vi "HXG2_PIDs_Array.vi"(0 "Calculated Values":T3, 1 "PID Cluster":T7, 2 "Evap Target Delta (-°F) 2":cluster{"m":dbl, "b":dbl}={"m"=0.2667, "b"=7.333}, 3 "AIR-LIQ Cluster":T4 {"Liq Cluster"."Liq TEMP %" min=0.0 max=100.0 step=1.0 format="%#.1f"; "Liq Cluster"."Liq FLOW %" min=0.0 max=100.0 step=1.0 format="%#.1f"; "Liq Cluster"."TLiq °F" min=40.0 max=180.0 step=1.0 format="%#.1f"; "Liq Cluster"."Mdot lbm/hr" min=0.0 max=1000.0 step=1.0 format="%#.1f"; "Air Cluster"."Air TEMP %" min=0.0 max=100.0 step=1.0 format="%#.1f"; "Air Cluster"."Air FLOW %" min=0.0 max=100.0 step=1.0 format="%#.1f"; "Air Cluster"."Tair  °F" min=-5.0 max=100.0 step=1.0 format="%#.1f"; "Air Cluster"."CFMs" min=0.0 max=200.0 step=1.0 format="%#.1f"}, 4 "Tank Target Delta (+°F)":dbl, 5 "error in (no error)":errorcluster, 6 "Analog In":T2, 7 "PID Ctrls":T1) -> (14 "PID Ctrls Out":T1, 19 "error out":errorcluster)   [LabVIEW 2012]
uses:
  Controls/HXG2_PIDctrlsOUT.ctl
  Controls/HXG2_PIDCluster.ctl
  Controls/HXG2_PIDon-off.ctl
  PID/HXG2_Horizontal PID Control.ctl
  PID/HXG2_Horizontal Reset Control.ctl
  Controls/HXG2_AirGly-Cluster.ctl
  Controls/UI/HXG2_UI_ControlSetAir.ctl
  Controls/UI/HXG2_UI_ControlSetGly.ctl
  Controls/HXG2_Calculated.ctl
  Controls/HXG2_AnalogIn.ctl
  Modules/EnableAirGly/HXG2enable.ctl
  Controls/UI/HXG2_NumDisplayLarge.ctl
  <vilib>/addons/control/pid/pid.llb/PID Advanced (DBL Array).vi
  <vilib>/addons/control/pid/pid.llb/PID Derivative Action Buffered (DBL Array).vi
  <vilib>/addons/control/pid/pid.llb/PID Get Advanced Error (DBL Array).vi
  <vilib>/addons/control/pid/pid.llb/PID Integral Action Buffered (DBL Array).vi
  <vilib>/addons/control/pid/pid.llb/PID Resize 1D Array.vi
  <vilib>/addons/control/pid/pid.llb/PID Get Advanced Error (DBL).vi
  <vilib>/addons/control/pid/pid.llb/PID Control Input Filter (DBL).vi
  <vilib>/addons/control/pid/pid.llb/PID Gain Schedule (DBL).vi
  <vilib>/addons/control/pid/pid.llb/PID Structure Conversion (DBL).vi
  <vilib>/addons/control/pid/pid.llb/PID Parameter Manager (DBL Array).vi
  <vilib>/addons/control/pid/NI_PID_pid.lvlib
panel:
  out "index out 2":i32
  out "index out":i32
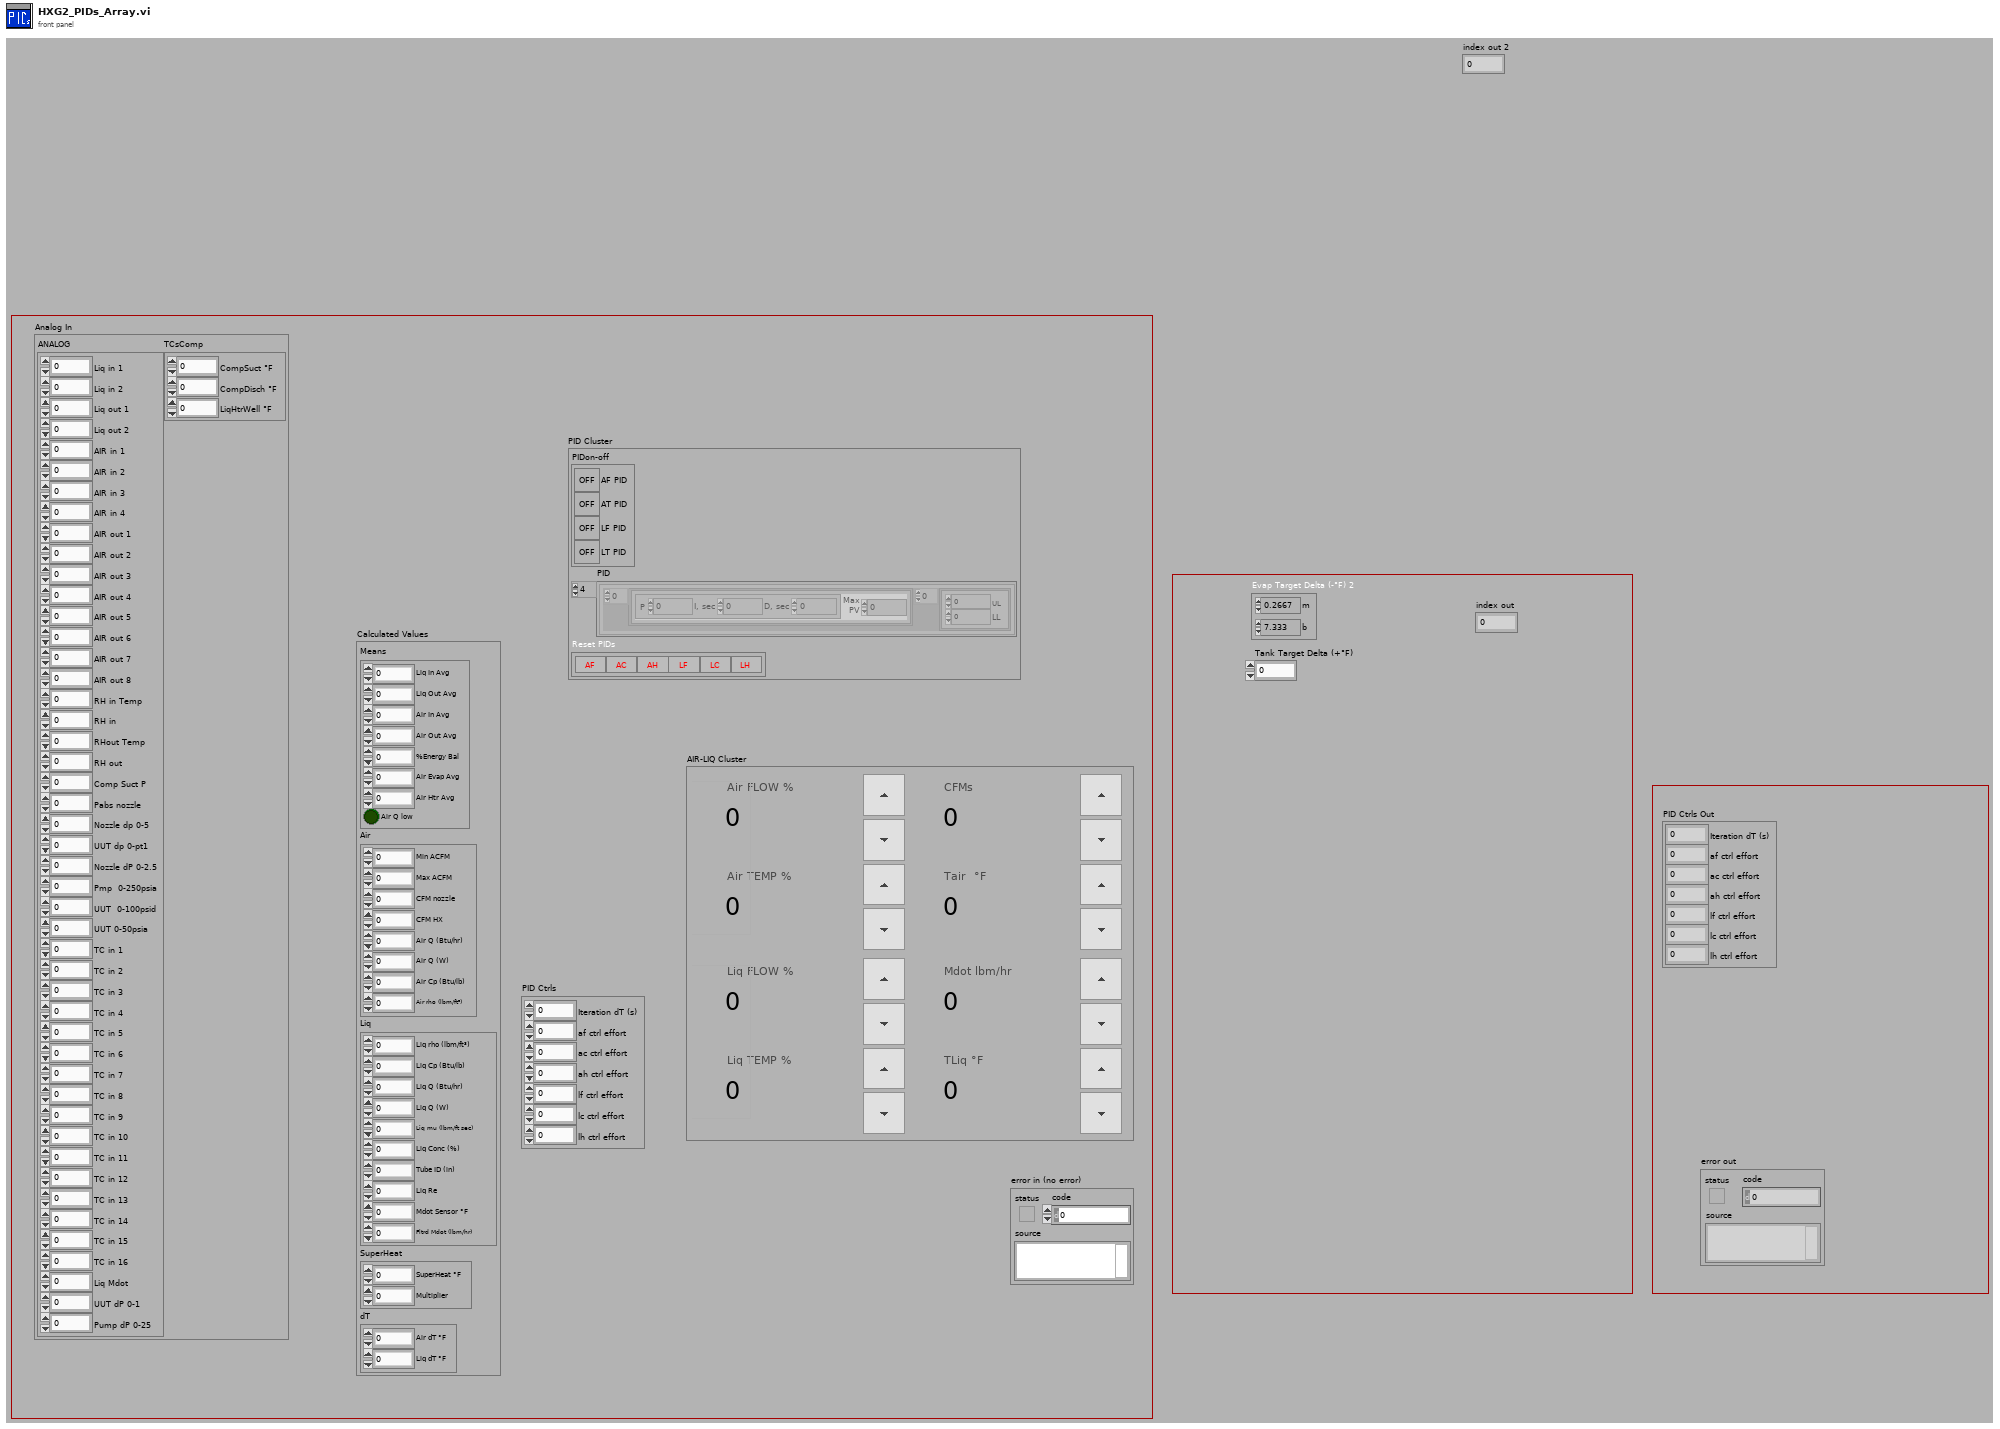
[diagram p1: front panel]
types:
  T1 = typedef "HXG2_PIDctrlsOUT.ctl" = cluster{"Iteration dT (s)":dbl, "af ctrl effort":dbl, "ac ctrl effort":dbl, "ah ctrl effort":dbl, "lf ctrl effort":dbl, "lc ctrl effort":dbl, "lh ctrl effort":dbl}
  T2 = typedef "HXG2_AnalogIn.ctl" = cluster{"ANALOG":cluster{"Liq in 1":dbl, "Liq in 2":dbl, "Liq out 1":dbl, "Liq out 2":dbl, "AIR in 1":dbl, "AIR in 2":dbl, "AIR in 3":dbl, "AIR in 4":dbl, "AIR out 1":dbl, "AIR out 2":dbl, "AIR out 3":dbl, "AIR out 4":dbl, "AIR out 5":dbl, "AIR out 6":dbl, "AIR out 7":dbl, "AIR out 8":dbl, "RH in Temp":dbl, "RH in":dbl, "RHout Temp":dbl, "RH out":dbl, "Comp Suct P":dbl, "Pabs nozzle":dbl, "Nozzle dp 0-5":dbl, "UUT dp 0-pt1":dbl, "Nozzle dP 0-2.5":dbl, "Pmp  0-250psia":dbl, "UUT  0-100psid":dbl, "UUT 0-50psia":dbl, "TC in 1":dbl, "TC in 2":dbl, "TC in 3":dbl, "TC in 4":dbl, "TC in 5":dbl, "TC in 6":dbl, "TC in 7":dbl, "TC in 8":dbl, "TC in 9":dbl, "TC in 10":dbl, "TC in 11":dbl, "TC in 12":dbl, "TC in 13":dbl, "TC in 14":dbl, "TC in 15":dbl, "TC in 16":dbl, "Liq Mdot":dbl, "UUT dP 0-1":dbl, "Pump dP 0-25":dbl}, "TCsComp":cluster{"CompSuct °F  ":dbl, "CompDisch °F":dbl, "LiqHtrWell °F":dbl}}
  T3 = typedef "HXG2_Calculated.ctl" = cluster{"Means":cluster{"Liq In Avg":dbl, "Liq Out Avg":dbl, "Air In Avg":dbl, "Air Out Avg":dbl, "%Energy Bal":dbl, "Air Evap Avg":dbl, "Air Htr Avg":dbl, "Air Q low":bool}, "Air":cluster{"Min ACFM":dbl, "Max ACFM":dbl, "CFM nozzle":dbl, "CFM HX":dbl, "Air Q (Btu/hr)":dbl, "Air Q (W)":dbl, "Air Cp (Btu/lb)":dbl, "Air rho (lbm/ft³)":dbl}, "Liq":cluster{"Liq rho (lbm/ft³)":dbl, "Liq Cp (Btu/lb)":dbl, "Liq Q (Btu/hr)":dbl, "Liq Q (W)":dbl, "Liq mu (lbm/ft sec)":dbl, "Liq Conc (%)":dbl, "Tube ID (in)":dbl, "Liq Re":dbl, "Mdot Sensor °F":dbl, "Fltrd Mdot (lbm/hr)":dbl}, "SuperHeat":cluster{"SuperHeat °F":dbl, "Multiplier":dbl}, "dT":cluster{"Air dT °F":dbl, "Liq dT °F":dbl}}
  T4 = typedef "HXG2_AirGly-Cluster.ctl" = cluster{"Air Cluster":T5, "Liq Cluster":T6}
  T5 = typedef "HXG2_UI_ControlSetAir.ctl" = cluster{"Air FLOW %":dbl, "Air TEMP % ":dbl, "CFMs":dbl, "Tair  °F":dbl}
  T6 = typedef "HXG2_UI_ControlSetGly.ctl" = cluster{"Liq FLOW %":dbl, "Liq TEMP % ":dbl, "Mdot lbm/hr":dbl, "TLiq °F":dbl}
  T7 = typedef "HXG2_PIDCluster.ctl" = cluster{"PIDon-off ":T8, "PID":T9, "Reset PIDs":T10}
  T8 = typedef "HXG2_PIDon-off.ctl" = cluster{"AF PID":bool, "AT PID":bool, "LF PID":bool, "LT PID":bool}
  T9 = typedef "HXG2_Horizontal PID Control.ctl" = cluster{"GainsArray":cluster{"Gains 2":cluster{"P":dbl, "I, sec":dbl, "D, sec":dbl}, "Max\nPV":dbl}[], "UL-LL Array":cluster{"UL":dbl, "LL  ":dbl}[]}[]
  T10 = typedef "HXG2_Horizontal Reset Control.ctl" = cluster{"AF":bool, "AC":bool, "AH":bool, "LF":bool, "LC":bool, "LH":bool}
  T11 = cluster{"setpoint high":dbl, "setpoint low":dbl}[]
  T12 = typedef "HXG2enable.ctl" = enum16{"Write Refs", "Write", "Pass"}
  T13 = enum16{"Academic (Standard)", "Parallel", "Series"}
  T14 = typedef "HXG2_NumDisplayLarge.ctl" = dbl
  T15 = cluster{"Gains 2":cluster{"P":dbl, "I, sec":dbl, "D, sec":dbl}, "Max\nPV":dbl}[]
  T16 = cluster{"proportional gain (Kc)":dbl, "integral time (Ti, min)":dbl, "derivative time (Td, min)":dbl}
  T17 = cluster{"output[0]":dbl, "output[1]":dbl, "output[2]":dbl}
  T18 = cluster{"[0]":dbl, "[1]":dbl, "[2]":dbl, "[3]":dbl}
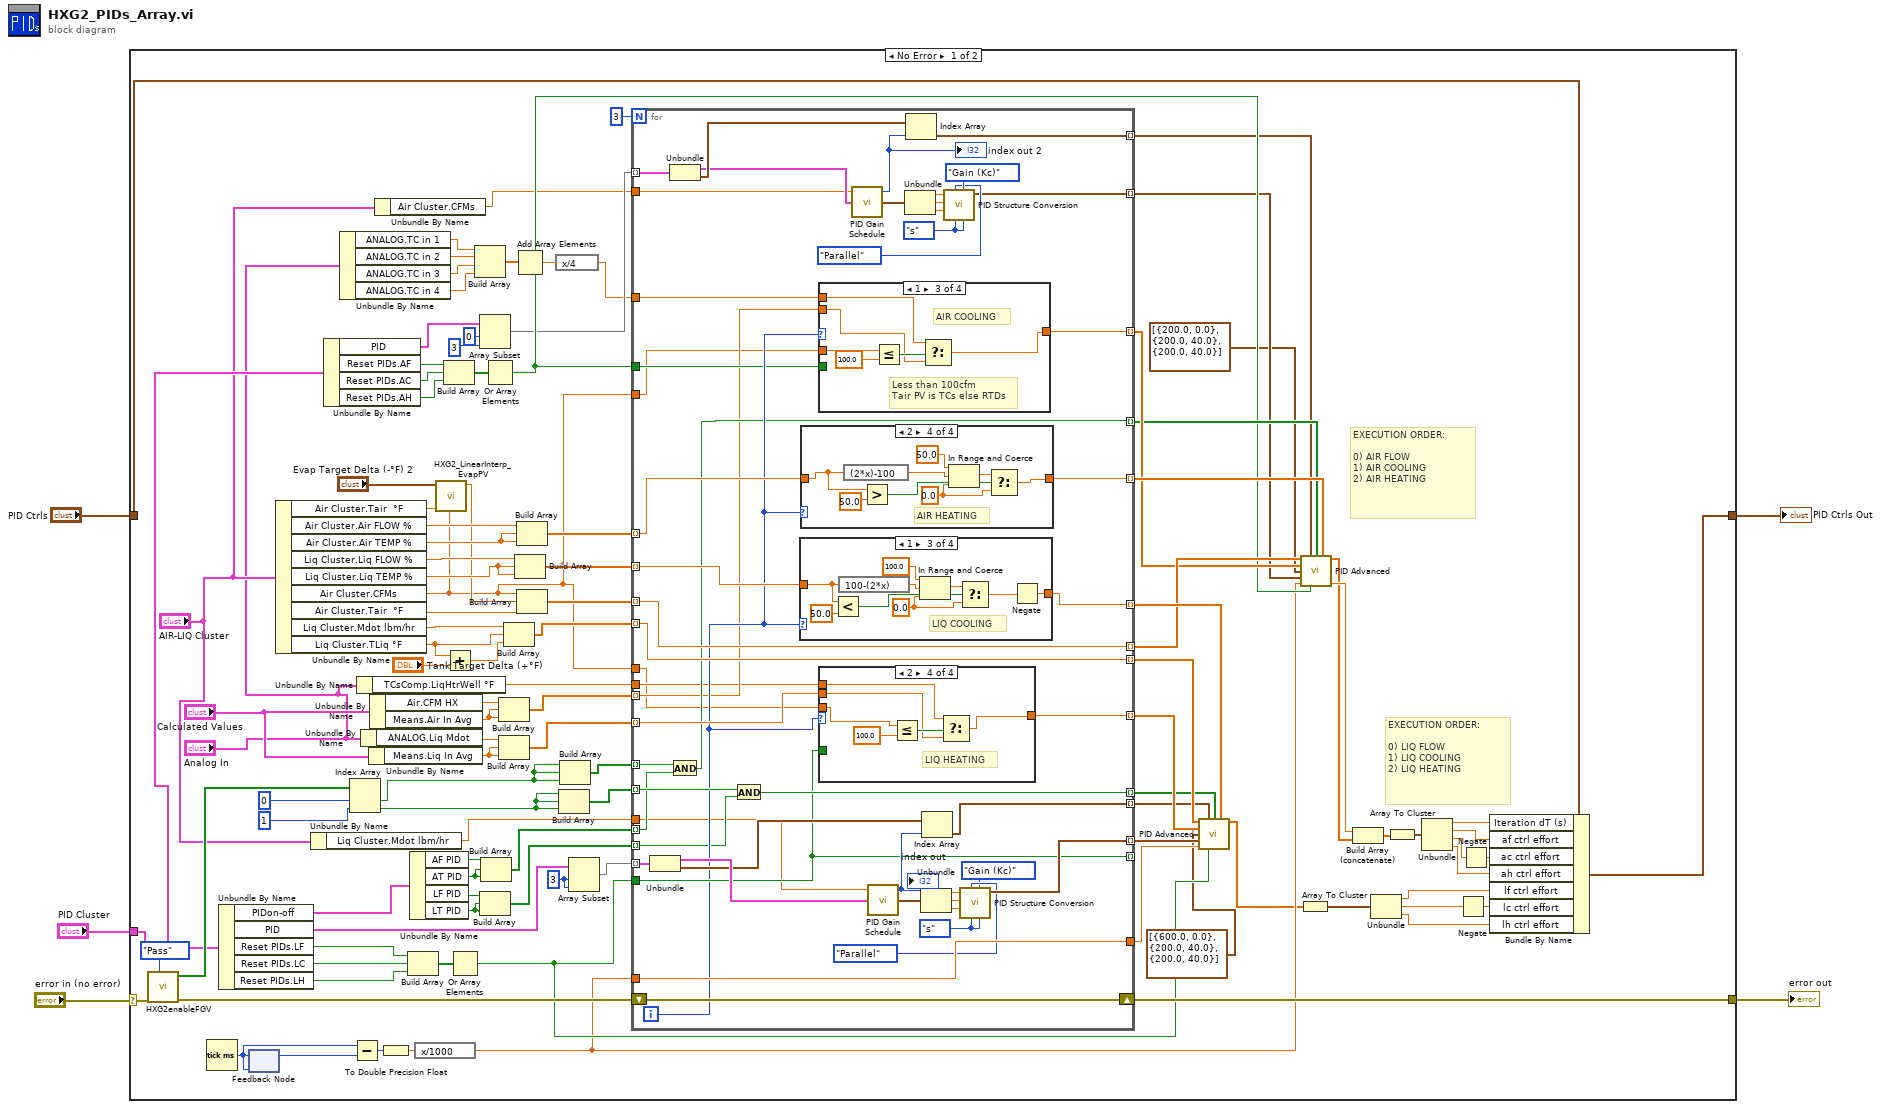
[diagram p0: block diagram]
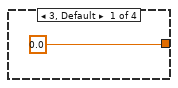
[diagram p2: hidden frame]
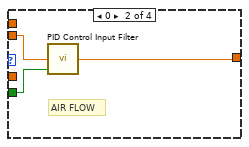
[diagram p3: hidden frame]
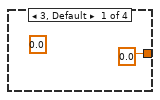
[diagram p5: hidden frame]
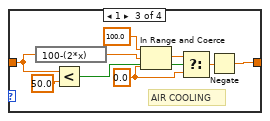
[diagram p7: hidden frame]
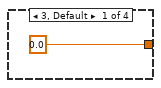
[diagram p8: hidden frame]
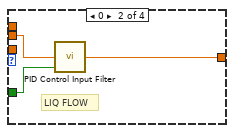
[diagram p9: hidden frame]
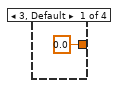
[diagram p11: hidden frame]
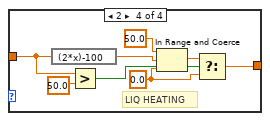
[diagram p13: hidden frame]
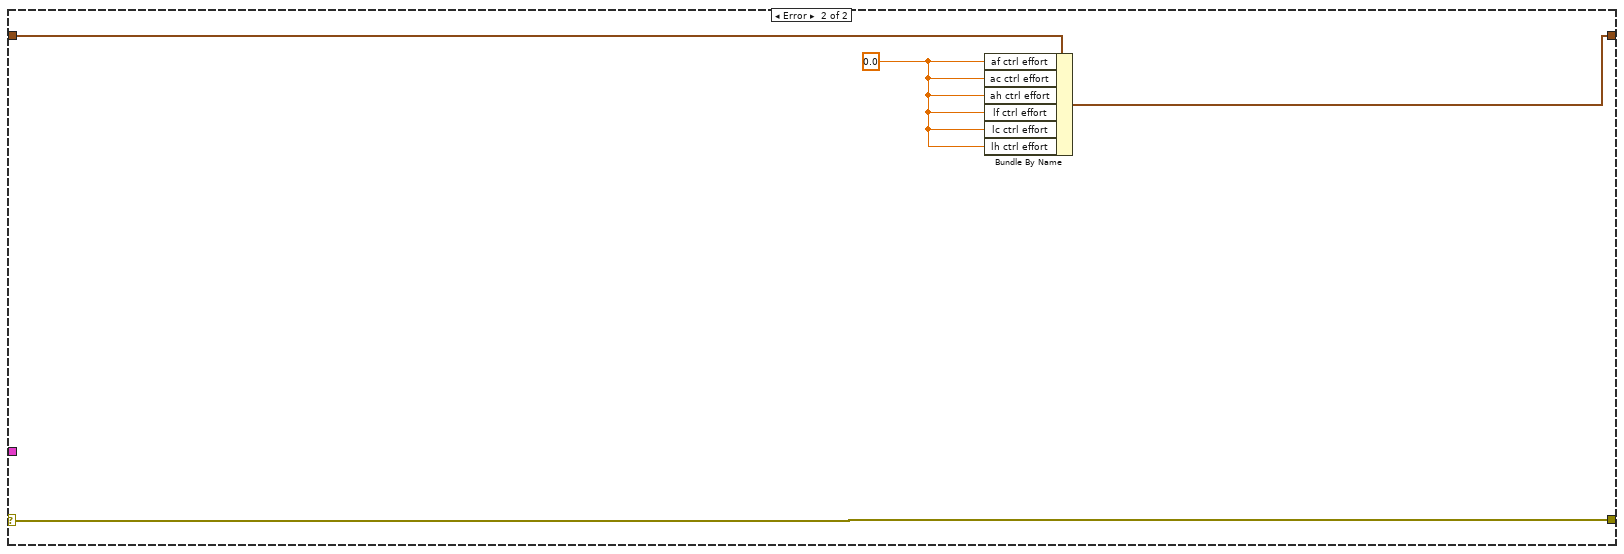
[diagram p14: hidden frame]
diagram:
  n1 = case shown="No Error" "error in (no error)" {
    selector: "error in (no error)" -> [w115 w232]
    tunnel: [w99 w232] -> w5
    tunnel: [w97 w230] -> w2
    tunnel: "PID Ctrls" -> [w98 w231]
    tunnel: "PID Cluster" -> [w61 _]
    frame No Error {
      w49 = 3 ("index")
      # "EXECUTION ORDER:\n\n0) AIR FLOW\n1) AIR COOLING\n2) AIR HEATING"
      # "EXECUTION ORDER:\n\n0) LIQ FLOW\n1) LIQ COOLING\n2) LIQ HEATING"
      n2 = call "HXG2enableFGV.vi"("ENABLE Ctrl"=HXG2enable."Pass", "error in (no error)"=w115) -> ("error out"=w100:errorcluster, "Air-Liq Out"=w102:bool[])  [unwired: 7 in, 1 out]
      n3 = Tick Count (ms)() -> (millisecond timer value=w108:u32)
      n4 = Unbundle By Name(w61) -> ("PIDon-off"=w94:T8, "PID"=w50:T9, "Reset PIDs.LF"=w56:bool, "Reset PIDs.LC"=w55:bool, "Reset PIDs.LH"=w54:bool)
      n5 = feedback #1(w108) -> (w106:u32)
      n6 = feedback-in #1(w108) -> ()
      n7 = Unbundle By Name("AIR-LIQ Cluster") -> ("Air Cluster.Tair  °F"=w8:dbl, "Air Cluster.Air FLOW %"=w84:dbl, "Air Cluster.Air TEMP %"=w83:dbl, "Liq Cluster.Liq FLOW %"=w112:dbl, "Liq Cluster.Liq TEMP %"=w111:dbl, "Air Cluster.CFMs"=w6:dbl, "Air Cluster.Tair  °F"=w15:dbl, "Liq Cluster.Mdot lbm/hr"=w26:dbl, "Liq Cluster.TLiq °F"=w13:dbl)
      n8 = Unbundle By Name("AIR-LIQ Cluster") -> ("Liq Cluster.Mdot lbm/hr"=w23:dbl)
      n9 = Unbundle By Name(w61) -> ("PID"=w46:T9, "Reset PIDs.AF"=w60:bool, "Reset PIDs.AC"=w59:bool, "Reset PIDs.AH"=w58:bool)
      n10 = Unbundle By Name("Analog In") -> ("ANALOG.TC in 1"=w22:dbl, "ANALOG.TC in 2"=w21:dbl, "ANALOG.TC in 3"=w20:dbl, "ANALOG.TC in 4"=w19:dbl)
      n11 = Index Array(array=w102, index #1=0 ("index"), index #2=1 ("index")) -> (element #1=w70:bool, element #2=w103:bool)
      n12 = Subtract(x=w108, y=w106) -> (x-y=w107:u32)
      n13 = Unbundle By Name("Analog In") -> ("TCsComp.LiqHtrWell °F"=w10:dbl)
      n14 = Unbundle By Name("Analog In") -> ("ANALOG.Liq Mdot"=w75:dbl)
      n15 = Unbundle By Name("Calculated Values") -> ("Means.Liq In Avg"=w74:dbl)
      n16 = Unbundle By Name("Calculated Values") -> ("Air.CFM HX"=w77:dbl, "Means.Air In Avg"=w76:dbl)
      n17 = Unbundle By Name("AIR-LIQ Cluster") -> ("Air Cluster.CFMs"=w25:dbl)
      n18 = To Double Precision Float(number=w107) -> (double precision float=w109:dbl)
      n19 = Build Array(w56, w55, w54) -> (w53:bool[])
      n20 = Unbundle By Name(w94) -> ("AF PID"=w66:bool, "AT PID"=w65:bool, "LF PID"=w67:bool, "LT PID"=w64:bool)
      n21 = expression code="x/1000"(w109) -> (w41:dbl)
      n22 = call "HXG2_LinearInterp_EvapPV.vi"("CFM"=w6, "Tair  °F"=w8, "Evap Target Delta (-°F) in"="Evap Target Delta (-°F) 2") -> ("Evap Target (F)"=w7:dbl)  [unwired: 8 in]
      n23 = Build Array(w60, w59, w58) -> (w57:bool[])
      n24 = Add(x=w13, y="Tank Target Delta (+°F)") -> (x+y=w12:dbl)
      n25 = Or Array Elements(Boolean array=w53) -> (logical OR=w52:bool)
      n26 = Build Array(w22, w21, w20, w19) -> (w18:dbl[])
      n27 = Array Subset(array=w46, index=0, length=3 ("index")) -> (w44:T9)
      n28 = Build Array(w67, w64, w64) -> (w63:bool[])
      n29 = Build Array(w66, w65, w65) -> (w62:bool[])
      n30 = Or Array Elements(Boolean array=w57) -> (logical OR=w51:bool)
      n31 = Build Array(w77, w76, w76) -> (w72:dbl[])
      n32 = Build Array(w75, w74, w74) -> (w73:dbl[])
      n33 = Build Array(w26, w13, w12) -> (w78:dbl[])
      n34 = Add Array Elements(numeric array=w18) -> (sum=w17:dbl)
      n35 = Build Array(w112, w111, w111) -> (w110:dbl[])
      n36 = Build Array(w84, w83, w83) -> (w82:dbl[])
      n37 = Build Array(w6, w7, w15) -> (w80:dbl[])
      n38 = expression code="x/4"(w17) -> (w16:dbl)
      n39 = Build Array(w103, w103, w103) -> (w101:bool[])
      n40 = Build Array(w70, w70, w70) -> (w69:bool[])
      n41 = Array Subset(array=w50, index=w49, length=w49) -> (w48:T9)
      n42 = for {
        N: 3 -> [_]
        tunnel: w63 -> [w140] mode=indexing
        tunnel: w73 -> [w159] mode=indexing
        tunnel: w78 -> [w155] mode=indexing
        tunnel: w110 -> [w165] mode=indexing
        tunnel: w41 -> [w150]
        tunnel: w101 -> [w168] mode=indexing
        tunnel: w48 -> [w167] mode=indexing
        shift-right: [w166] -> w99
        shift-left: w100 -> [w166]
        tunnel: w52 -> [w149]
        tunnel: [w155] -> w93 mode=indexing
        tunnel: [w154] -> w92 mode=indexing
        tunnel: [w153] -> w91 mode=indexing
        tunnel: [w152] -> w90 mode=indexing
        tunnel: [w146] -> w89 mode=indexing
        tunnel: [w151] -> w88 mode=indexing
        tunnel: [w150] -> w87
        tunnel: [w149] -> _ mode=indexing
        tunnel: w82 -> [w145] mode=indexing
        tunnel: [w144] -> w81 mode=indexing
        tunnel: w80 -> [w143] mode=indexing
        tunnel: [w143] -> w79 mode=indexing
        tunnel: w72 -> [w124] mode=indexing
        tunnel: [w142] -> w71 mode=indexing
        tunnel: w69 -> [w139] mode=indexing
        tunnel: [w138] -> w68 mode=indexing
        tunnel: w62 -> [w137] mode=indexing
        tunnel: w51 -> [w136]
        tunnel: w44 -> [w127] mode=indexing
        tunnel: [w123] -> w43 mode=indexing
        tunnel: [w122] -> w42 mode=indexing
        tunnel: w25 -> [w121]
        tunnel: w23 -> [w120]
        tunnel: w16 -> [w119]
        tunnel: w10 -> [w118]
        tunnel: w6 -> [w117]
        tunnel: w6 -> [w116]
        i -> [w141]
        w132 = enum16{"min", "s"}."s" ("integral unit")
        w160 = enum16{"min", "s"}."s" ("integral unit")
        n43 = Unbundle(w167) -> ("GainsArray"=w157:T15, "UL-LL Array"=w156:cluster{"UL":dbl, "LL  ":dbl}[])
        n44 = Unbundle(w127) -> ("GainsArray"=w125:T15, "UL-LL Array"=w126:cluster{"UL":dbl, "LL  ":dbl}[])
        n45 = And(x=w139, y=w137) -> (x .and. y?=w138:bool)
        n46 = And(x=w168, y=w140) -> (x .and. y?=w152:bool)
        n47 = case shown="1" w141 {
          tunnel: w165 -> [_ w211 w213 w223]
          tunnel: [0.0 ("Liq In Avg") w211 w212 w221] -> w153
          frame 3, Default {
          }
          frame 0 {
            # "LIQ FLOW"
          }
          frame 1 {
            w216 = T14 0.0 ("lower limit")
            # "LIQ COOLING"
            n48 = Less?(x=w213, y=T14 50.0) -> (x < y?=w215:bool)
            n49 = expression code="100-(2*x)"(w213) -> (w218:dbl)
            n50 = In Range and Coerce(upper limit=T14 100.0, x=w218, lower limit=w216) -> (coerced(x)=w219:T14)  [unwired: 1 out]
            n51 = Select(t=w219, s=w215, f=w216) -> (s? t:f=w220:T14)
            n52 = Negate(x=w220) -> (-x=w212:T14)
          }
          frame 2 {
            w228 = T14 0.0 ("lower limit")
            # "LIQ HEATING"
            n53 = expression code="(2*x)-100"(w223) -> (w226:dbl)
            n54 = Greater?(x=w223, y=T14 50.0) -> (0:w224:bool)
            n55 = In Range and Coerce(upper limit=T14 50.0, x=w226, lower limit=w228) -> (coerced(x)=w227:T14)  [unwired: 1 out]
            n56 = Select(t=w227, s=w224, f=w228) -> (s? t:f=w221:T14)
          }
        }
        n57 = case shown="2" w141 {
          tunnel: w145 -> [_ w181 w184 w193]
          tunnel: [0.0 ("Liq In Avg") w181 w182 w191] -> w144
          frame 3, Default {
            (unwired) 0.0 ("Liq In Avg")
          }
          frame 0 {
            # "AIR FLOW"
          }
          frame 1 {
            w186 = T14 0.0 ("lower limit")
            # "AIR COOLING"
            n58 = expression code="100-(2*x)"(w184) -> (w187:dbl)
            n59 = Less?(x=w184, y=T14 50.0) -> (x < y?=w185:bool)
            n60 = In Range and Coerce(upper limit=T14 100.0, x=w187, lower limit=w186) -> (coerced(x)=w188:T14)  [unwired: 1 out]
            n61 = Select(t=w188, s=w185, f=w186) -> (s? t:f=w190:T14)
            n62 = Negate(x=w190) -> (-x=w182:T14)
          }
          frame 2 {
            w198 = T14 0.0 ("lower limit")
            # "AIR HEATING"
            n63 = expression code="(2*x)-100"(w193) -> (w196:dbl)
            n64 = Greater?(x=w193, y=T14 50.0) -> (0:w194:bool)
            n65 = In Range and Coerce(upper limit=T14 50.0, x=w196, lower limit=w198) -> (coerced(x)=w197:T14)  [unwired: 1 out]
            n66 = Select(t=w197, s=w194, f=w198) -> (s? t:f=w191:T14)
          }
        }
        n67 = case shown="1" w141 {
          tunnel: w124 -> [_ w172 w175 w179]
          tunnel: [0.0 ("Liq In Avg") w171 w173 w179] -> w142
          tunnel: w136 -> [_ w170 _ _]
          tunnel: w119 -> [_ _ w174 _]
          tunnel: w117 -> [_ _ w178 _]
          frame 3, Default {
          }
          frame 0 {
            # "AIR FLOW"
            n68 = call-poly <vilib>:"PID Control Input Filter.vi"("reinitialize? (F)"=w170, "input"=w172) -> ("output"=w171:dbl)  [unwired: 3 in]
          }
          frame 1 {
            # "Less than 100cfm\nTair PV is TCs else RTDs"
            # "AIR COOLING"
            n69 = Less Or Equal?(x=w178, y=100.0) -> (x <= y?=w176:bool)
            n70 = Select(t=w174, s=w176, f=w175) -> (s? t:f=w173:dbl)
          }
          frame 2 {
            # "AIR HEATING"
          }
        }
        n71 = case shown="2" w141 {
          tunnel: w159 -> [_ w202 w203 w206]
          tunnel: [0.0 ("Liq In Avg") w200 w203 w204] -> w154
          tunnel: w149 -> [_ w201 _ _]
          tunnel: w118 -> [_ _ _ w205]
          tunnel: w116 -> [_ _ _ w207]
          frame 3, Default {
          }
          frame 0 {
            # "LIQ FLOW"
            n72 = call-poly <vilib>:"PID Control Input Filter.vi"("reinitialize? (F)"=w201, "input"=w202) -> ("output"=w200:dbl)  [unwired: 3 in]
          }
          frame 1 {
            # "LIQ COOLING"
          }
          frame 2 {
            # "LIQ HEATING"
            n73 = Less Or Equal?(x=w207, y=100.0) -> (x <= y?=w209:bool)
            n74 = Select(t=w205, s=w209, f=w206) -> (s? t:f=w204:dbl)
          }
        }
        n75 = call-poly <vilib>:"PID Gain Schedule.vi"("PID gain schedule"=w125, "gain scheduling value"=w121) -> ("PID gains out"=w128:T16, "index out"=w133:i32)  [unwired: 2 in]
        "index out 2" <- w133
        n76 = call-poly <vilib>:"PID Gain Schedule.vi"("PID gain schedule"=w157, "gain scheduling value"=w120) -> ("PID gains out"=w164:T16, "index out"=w158:i32)  [unwired: 2 in]
        "index out" <- w158
        n77 = Unbundle(w128) -> ("proportional gain (Kc)"=w129:dbl, "integral time (Ti, min)"=w130:dbl, "derivative time (Td, min)"=w131:dbl)
        n78 = Index Array(array=w126, index=w133) -> (element=w122:cluster{"UL":dbl, "LL  ":dbl})
        n79 = Unbundle(w164) -> ("proportional gain (Kc)"=w163:dbl, "integral time (Ti, min)"=w162:dbl, "derivative time (Td, min)"=w161:dbl)
        n80 = Index Array(array=w156, index=w158) -> (element=w146:cluster{"UL":dbl, "LL  ":dbl})
        n81 = call-poly <vilib>:"PID Structure Conversion.vi"("derivative unit"=w132, "proportional unit"=enum16{"Gain (Kc)", "Band (PB)"}."Gain (Kc)", "integral unit"=w132, "PID structure"=T13."Parallel", "derivative"=w131, "integral"=w130, "proportional"=w129) -> ("PID gains"=w123:T16)  [unwired: 4 in]
        n82 = call-poly <vilib>:"PID Structure Conversion.vi"("derivative unit"=w160, "proportional unit"=enum16{"Gain (Kc)", "Band (PB)"}."Gain (Kc)", "integral unit"=w160, "PID structure"=T13."Parallel", "derivative"=w161, "integral"=w162, "proportional"=w163) -> ("PID gains"=w151:T16)  [unwired: 4 in]
      }
      n83 = call-poly <vilib>:"PID Advanced.vi"("setpoint"=w93, "output range"=w89, "auto? (T)"=w90, "manual control"=w91, "process variable"=w92, "setpoint range"=T11 [{"setpoint high"=600.0, "setpoint low"=0.0}, {"setpoint high"=200.0, "setpoint low"=40.0}, {"setpoint high"=200.0, "setpoint low"=40.0}], "PID gains"=w88, "dt (s)"=w87, "reinitialize? (F)"=w52) -> ("output"=w40:dbl[])  [unwired: 5 in, 1 out]
      n84 = Array To Cluster(array=w40) -> (cluster=w96:T17)
      n85 = call-poly <vilib>:"PID Advanced.vi"("setpoint"=w79, "output range"=w42, "auto? (T)"=w68, "manual control"=w81, "process variable"=w71, "setpoint range"=T11 [{"setpoint high"=200.0, "setpoint low"=0.0}, {"setpoint high"=200.0, "setpoint low"=40.0}, {"setpoint high"=200.0, "setpoint low"=40.0}], "PID gains"=w43, "dt (s)"=w41, "reinitialize? (F)"=w51) -> ("output"=w35:dbl[], "dt out (s)"=w36:dbl)  [unwired: 5 in]
      n86 = Build Array (concatenate)(w36, w35) -> (w34:dbl[])
      n87 = Unbundle(w96) -> ("output[0]"=w39:dbl, "output[1]"=w38:dbl, "output[2]"=w37:dbl)
      n88 = Array To Cluster(array=w34) -> (cluster=w33:T18)
      n89 = Unbundle(w33) -> ("[0]"=w32:dbl, "[1]"=w31:dbl, "[2]"=w30:dbl, "[3]"=w29:dbl)
      n90 = Negate(x=w38) -> (-x=w85:dbl)
      n91 = Negate(x=w30) -> (-x=w95:dbl)
      n92 = Bundle By Name(cluster=w98, "Iteration dT (s)"=w32, "af ctrl effort"=w31, "ac ctrl effort"=w95, "ah ctrl effort"=w29, "lf ctrl effort"=w39, "lc ctrl effort"=w85, "lh ctrl effort"=w37) -> (w97:T1)
    }
    frame Error {
      w229 = 0.0 ("af ctrl effort")
      n93 = Bundle By Name(cluster=w231, "af ctrl effort"=w229, "ac ctrl effort"=w229, "ah ctrl effort"=w229, "lf ctrl effort"=w229, "lc ctrl effort"=w229, "lh ctrl effort"=w229) -> (w230:T1)
    }
  }
  "error out" <- w5
  "PID Ctrls Out" <- w2
